vi "Auto Class Name.vi"(7 "QD Launch VI Panel?":bool, 8 "error in (no error)":errorcluster, 11 "VI in":refnum<vi>) -> (0 "error out":errorcluster, 3 "VI out":refnum<vi>, 4 "Completed":bool)   [LabVIEW 2017]
uses:
  <vilib>/regexp/Match Regular Expression.xnode
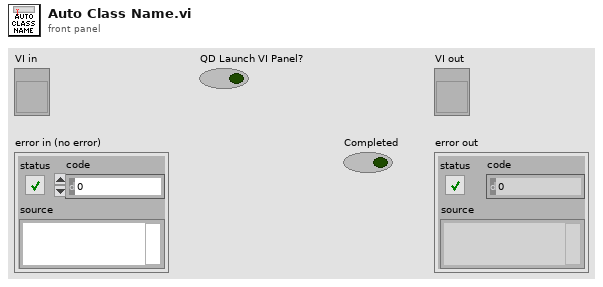
[diagram p1: front panel]
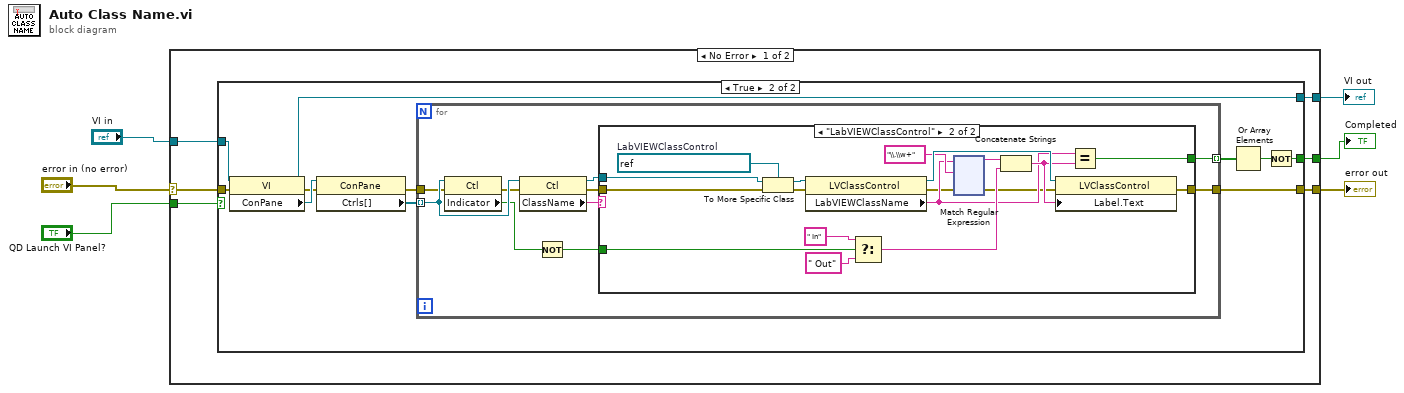
[diagram p0: block diagram]
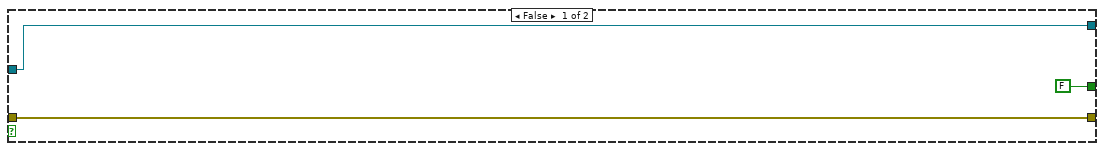
[diagram p2: hidden frame]
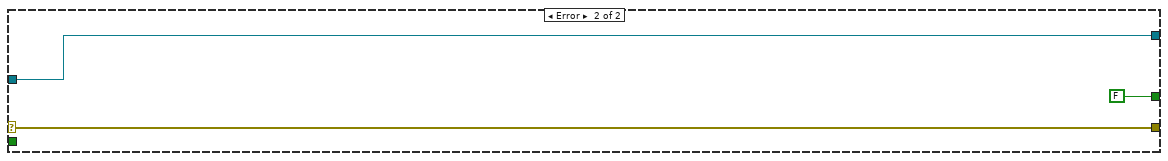
[diagram p4: hidden frame]
diagram:
  n1 = case shown="No Error" "error in (no error)" {
    selector: "error in (no error)" -> [w10 w172]
    tunnel: [w12 FALSE] -> w6
    tunnel: "VI in" -> [w11 w171]
    tunnel: [w9 w172] -> w3
    tunnel: [w8 w171] -> w2
    tunnel: "QD Launch VI Panel?" -> [w7 _]
    frame No Error {
      n2 = case shown="True" w7 {
        tunnel: [FALSE w22] -> w12
        tunnel: w11 -> [w15 w21]
        tunnel: w10 -> [w14 w20]
        tunnel: [w14 w17] -> w9
        tunnel: [w15 w16] -> w8
        frame False {
        }
        frame True {
          n3 = property class="VI"(reference=w21, error in=w20) -> (reference out=w16:refnum<vi>, error out=w19:errorcluster, "ConPane"=w25:refnum<vi>)
          n4 = property class="ConPane"(reference=w25, error in=w19) -> (error out=w18:errorcluster, "Ctrls[]"=w26:refnum<vi>[])  [unwired: 1 out]
          n5 = for {
            tunnel: w26 -> [w34] mode=indexing
            tunnel: [w31] -> w24 mode=indexing
            tunnel: w18 -> [w30]
            tunnel: [w27] -> w17
            n6 = property class="Ctl"(reference=w34, error in=w30) -> (error out=w29:errorcluster, "Indicator"=w33:bool)  [unwired: 1 out]
            n7 = property class="Ctl"(reference=w34, error in=w29) -> (reference out=w35:refnum<vi>, error out=w28:errorcluster, "ClassName"=w36:string)
            n8 = Not(x=w33) -> (.not. x?=w32:bool)
            n9 = case shown="\"LabVIEWClassControl\"" w36 {
              tunnel: w35 -> [_ w55]
              tunnel: w32 -> [_ w45]
              tunnel: [_ w42] -> w31
              tunnel: w28 -> [w37 w41]
              tunnel: [w37 w38] -> w27
              frame "False", Default {
              }
              frame "LabVIEWClassControl" {
                w54 = refnum<vi> refnum  # LabVIEWClassControl
                n10 = To More Specific Class(target class=w54, reference=w55, error in=w41) -> (specific class reference=w53:refnum<vi>, error out=w52:errorcluster)
                n11 = property class="LVClassControl"(reference=w53, error in=w52) -> (reference out=w51:refnum<vi>, error out=w40:errorcluster, "LabVIEWClassName"=w43:string)
                n12 = Select(t=" In", s=w45, f=" Out") -> (s? t:f=w49:string)
                n13 = xnode "Match Regular Expression"("input string"=w43, "regular expression"="\\.\\w+", "error in"=w40) -> ("before match"=w46:string, "error out"=w39:errorcluster)  [unwired: 3 in, 3 out]
                n14 = Concatenate Strings(w46, w49) -> (w44:string)
                n15 = property class="LVClassControl"(reference=w51, error in=w39, "Label.Text"=w44) -> (error out=w38:errorcluster)  [unwired: 1 out]
                n16 = Equal?(x=w43, y=w44) -> (x = y?=w42:bool)
              }
            }
          }
          n17 = Or Array Elements(Boolean array=w24) -> (logical OR=w23:bool)
          n18 = Not(x=w23) -> (.not. x?=w22:bool)
        }
      }
    }
    frame Error {
    }
  }
  "Completed" <- w6
  "error out" <- w3
  "VI out" <- w2
